vi "Test_LaunchActors_CallerError_EmergencyStopNested.vi"(8 "error in (no error)":errorcluster, 11 "TestCase in":refnum<class "TestLaunchAndShutdown.lvclass">) -> (0 "error out":errorcluster, 3 "TestCase out":refnum<class "TestLaunchAndShutdown.lvclass">)   [LabVIEW 2017, in "TestLaunchAndShutdown.lvclass"]
uses:
  TestLaunchAndShutdown.lvclass
  <vilib>/ActorFramework/Actor/Actor.lvclass
  <vilib>/ActorFramework/Report Error Msg/Report Error Msg.lvclass/Report Error Msg.ctl
  <vilib>/ActorFramework/Message Enqueuer/Message Enqueuer.lvclass/Message Enqueuer.ctl
  <vilib>/ActorFramework/Message Enqueuer/Enqueue.vi
  Doubles/ActorNotifiesWhenStopped/ActorNotifiesWhenStopped.lvclass
  C:/Program Files (x86)/National Instruments/LabVIEW 2017/vi.lib/ActorFramework/Actor/Actor.lvclass
  <vilib>/ActorFramework/Report Error Msg/Report Error Msg.lvclass
  C:/Program Files (x86)/National Instruments/LabVIEW 2017/vi.lib/ActorFramework/Message/Message.lvclass
  <vilib>/ActorFramework/Message Priority Queue/Priority Enqueue.vi
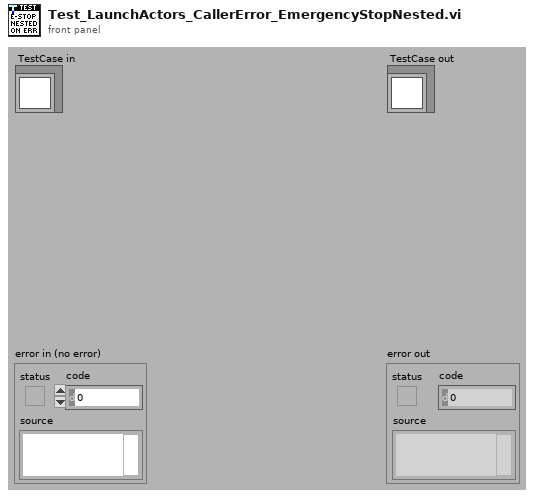
[diagram p1: front panel]
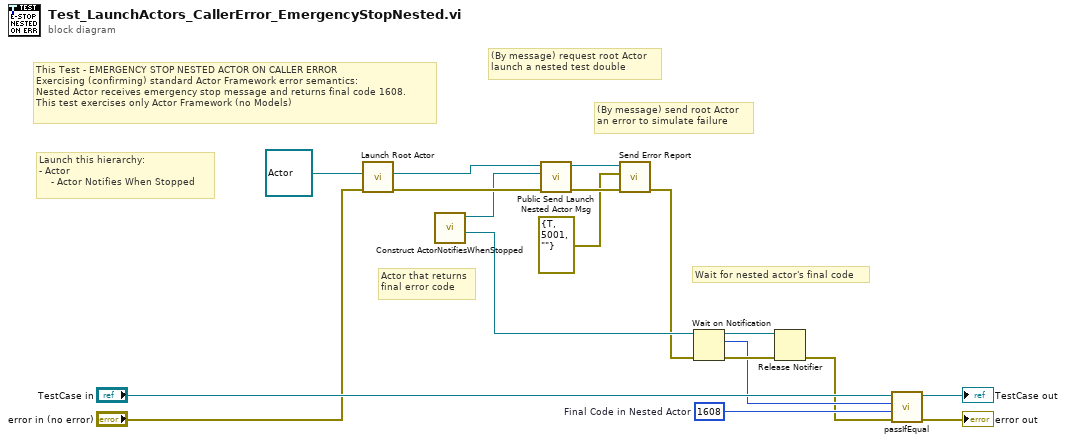
[diagram p0: block diagram]
diagram:
  w9 = 1608  # Final Code in Nested Actor
  # "(By message) send root Actor\nan error to simulate failure"
  # "(By message) request root Actor\nlaunch a nested test double"
  # "Wait for nested actor's final code"
  # "This Test - EMERGENCY STOP NESTED ACTOR ON CALLER ERROR\nExercising (confirming) standard Actor Framework error semantics:\nNested Actor receives emergency stop message and returns final code 1608.\nThis test exercises only Actor Framework (no Models)"
  # "Actor that returns\nfinal error code"
  # "Launch this hierarchy:\n- Actor\n    - Actor Notifies When Stopped"
  n1 = call <vilib>:"Launch Root Actor.vi"("error in (no error)"="error in (no error)", "Actor"=refnum<class "Actor.lvclass"> refnum) -> ("error out"=w14:errorcluster, "Actor's Enqueuer"=w11:refnum<class "Message Enqueuer.lvclass">)  [unwired: 8 in]
  n2 = call "Construct ActorNotifiesWhenStopped.vi"() -> ("Final Error Notifier"=w5:refnum<notifier>, "RootModelNotifiesWhenStopped out"=w6:refnum<class "ActorNotifiesWhenStopped.lvclass">)  [unwired: 10 in]
  n3 = call "Public Send Launch Nested Actor Msg.vi"("error in"=w14, "Nested Actor"=w6, "Self Enqueuer in"=w11) -> ("error out"=w4:errorcluster, "Self Enqueuer out"=w2:refnum<class "Message Enqueuer.lvclass">)  [unwired: 7 in]
  n4 = call <vilib>:"Send Error Report.vi"("error in (no error)"=w4, "Error From Sender"=errorcluster {"status"=TRUE, "code"=5001, "source"=""}, "Message Enqueuer"=w2) -> ("error out"=w3:errorcluster)  [unwired: 8 in]
  n5 = Wait on Notification(notifier=w5, error in (no error)=w3) -> (notifier out=w12:refnum<notifier>, notification=w10:i32, error out=w13:errorcluster)  [unwired: 2 in, 1 out]
  n6 = Release Notifier(notifier=w12, error in (no error)=w13) -> (error out=w8:errorcluster)  [unwired: 1 in, 2 out]
  n7 = call-dynamic "passIfEqual.vi"("error in (no error)"=w8, "y"=w9, "x"=w10, "TestCase in"="TestCase in") -> ("error out"=→"error out":errorcluster, "TestCase out"=→"TestCase out":refnum<class "TestLaunchAndShutdown.lvclass">)  [unwired: 6 in]
